vi "SaveToLVSET.vi"(6 "Save?":bool, 7 "Overwrite Existing Default Settings?":bool, 8 "Error In":errorcluster, 11 "System Paramters For Each Module":T1[](array[typedef]) {"sync_freq_div" items=["1"=1, "2"=2, "4"=4]; "cfd_zc_level" min=-96 max=96 step=0.1 format="%#_3g"; "cfd_limit_low" min=-500 max=0 step=0.1 format="%#_3g"; "sync_zc_level" min=-96 max=96 step=0.1 format="%#_3g"; "sync_threshold" min=-500 max=-20 step=0.1 format="%#_3g"; "tac_limit_low" format="%.3g"; "tac_limit_high" min=0 max=100 step=0.1 format="%.3g"; "collect_time" min=1e-07 max=100000 step=0.001; "tac_offset" min=0 max=100 step=0.1 format="%.4g"; "tac_gain" min=1 max=15 step=1; "tac_range" format="%^#_6g"}) -> (0 "Error Out":errorcluster)   [LabVIEW 2017]
doc: "This convenience VI stores the given system parameters into a LVSET file. The default file which is also used as the file to store the last used settings for each module is located in \"C:\\BHdata\\SPCM\\SPCDefaultVal.lvset\". \nThe user has the choice to overwrite this file or to use another file location to store the settings. \n\ninfo@becker-hickl.com"
uses:
  Example_Controls/UserInput.ctl
panel:
  in  "Saving Path":path=path "C:/BHdata/SPCM/SPCDefaultVal.lvset"
  # "TAC / Time Range"
  # "CFD"
  # "(start)"
  # "SYNC"
  # "(stop)"
  # "range"
  # "gain"
  # "threshold(LL)"
  # "offset"
  # "limit high"
  # "limit low"
  # "zero cross(ZC)"
  # "Collection Time"
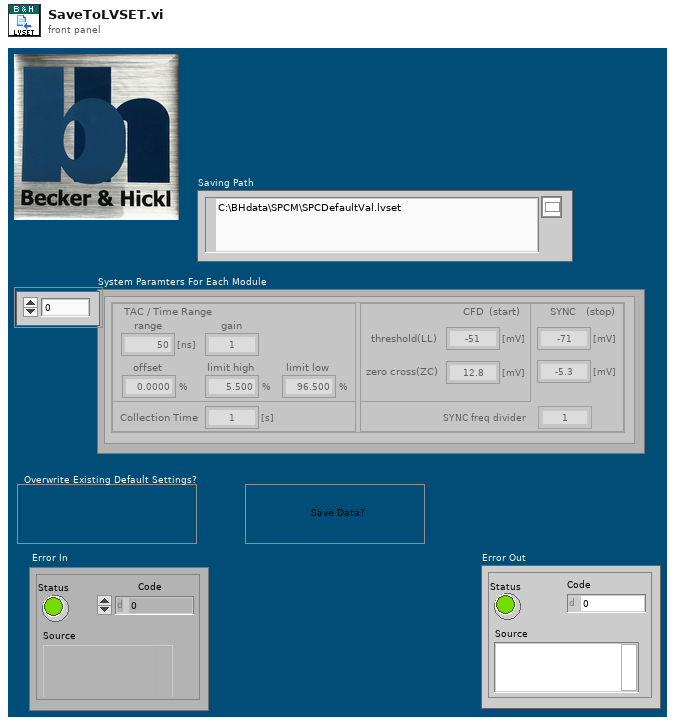
[diagram p1: front panel]
types:
  T1 = typedef "UserInput.ctl" = cluster{"tac_range":sgl, "tac_gain":i16, "tac_offset":sgl, "tac_limit_high":sgl, "tac_limit_low":sgl, "collect_time":sgl, "sync_threshold":sgl, "sync_zc_level":sgl, "sync_freq_div":i16, "cfd_limit_low":sgl, "cfd_zc_level":sgl}
  T2 = enum16{"big-endian, network order", "native, host order", "little-endian"}
  T3 = enum16{"open", "replace", "create", "open or create", "replace or create", "replace or create with confirmation"}
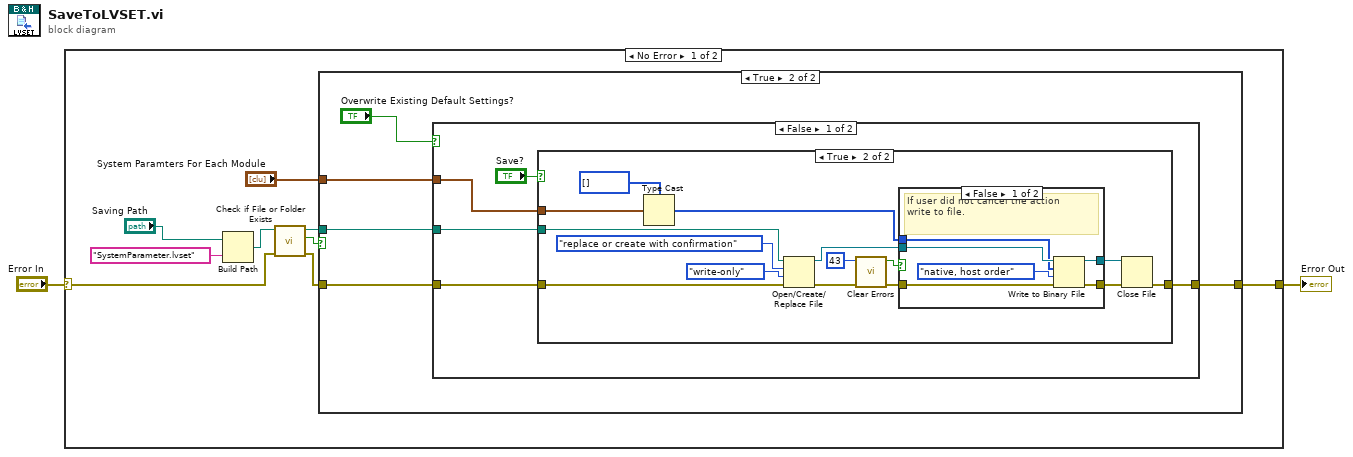
[diagram p0: block diagram]
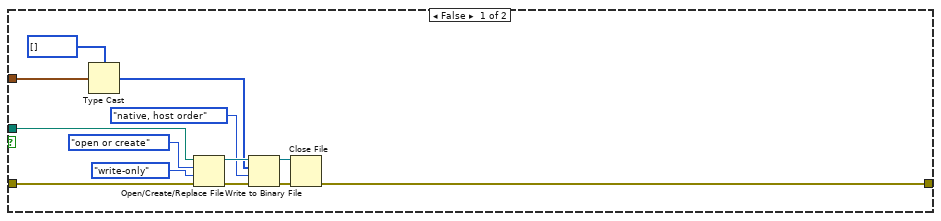
[diagram p2: hidden frame]
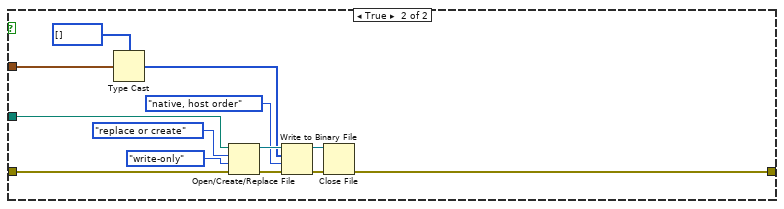
[diagram p5: hidden frame]
diagram:
  n1 = case shown="No Error" "Error In" {
    selector: "Error In" -> [w4 w72]
    tunnel: [w8 w72] -> w2
    frame No Error {
      n2 = Build Path(base path="Saving Path", name or relative path="SystemParameter.lvset") -> (appended path=w5:path)
      n3 = call <vilib>:"Check if File or Folder Exists.vi"("error in (no error)"=w4, "path"=w5) -> ("error out"=w3:errorcluster, "file or folder exists?"=w10:bool, "dup path"=w11:path)  [unwired: 7 in]
      n4 = case shown="True" w10 {
        tunnel: w11 -> [w24 w29]
        tunnel: w3 -> [w23 w28]
        tunnel: [w22 w27] -> w8
        tunnel: "System Paramters For Each Module" -> [w15 w26]
        frame False {
          n5 = Type Cast(type=u8[] [], x=w15) -> (*(type *) &x=w13:u8[])
          n6 = Open/Create/Replace File(file path (use dialog)=w24, error in=w23, operation (0:open)=T3."open or create", access (0:read/write)=enum16{"read/write", "read-only", "write-only"}."write-only") -> (refnum out=w19:refnum<file>, error out=w18:errorcluster)  [unwired: 2 in, 1 out]
          n7 = Write to Binary File(file (use dialog)=w19, data=w13, error in=w18, 9:T2."native, host order" ("byte order (0:big-endian, network order)")) -> (refnum out=w17:refnum<file>, error out=w16:errorcluster)  [unwired: 2 in, 1 out]
          n8 = Close File(refnum=w17, error in=w16) -> (error out=w22:errorcluster)  [unwired: 1 out]
        }
        frame True {
          n9 = case shown="False" "Overwrite Existing Default Settings?" {
            tunnel: w29 -> [w30 w71]
            tunnel: w28 -> [w34 w68]
            tunnel: [w32 w63] -> w27
            tunnel: w26 -> [w33 w60]
            frame False {
              n10 = case shown="True" "Save?" {
                tunnel: w34 -> [w35 w42]
                tunnel: w33 -> [_ w41]
                tunnel: [w35 w40] -> w32
                tunnel: w30 -> [_ w39]
                frame False {
                }
                frame True {
                  n11 = Type Cast(type=u8[] [], x=w41) -> (*(type *) &x=w46:u8[])
                  n12 = Open/Create/Replace File(file path (use dialog)=w39, error in=w42, operation (0:open)=T3."replace or create with confirmation", access (0:read/write)=enum16{"read/write", "read-only", "write-only"}."write-only") -> (refnum out=w50:refnum<file>, error out=w49:errorcluster)  [unwired: 2 in, 1 out]
                  n13 = call <vilib>:"Clear Errors.vi"("error in (no error)"=w49, "specific error code to clear (0: all)"=43) -> ("error out"=w38:errorcluster, "specific error cleared?"=w36:bool)  [unwired: 4 in]
                  n14 = case shown="False" w36 {
                    tunnel: w50 -> [w56 w58]
                    tunnel: w38 -> [w55 w57]
                    tunnel: [w54 w58] -> w48
                    tunnel: [w53 w57] -> w47
                    tunnel: w46 -> [w52 _]
                    frame False {
                      # "If user did not cancel the action\nwrite to file."
                      n15 = Write to Binary File(file (use dialog)=w56, data=w52, error in=w55, 9:T2."native, host order" ("byte order (0:big-endian, network order)")) -> (refnum out=w54:refnum<file>, error out=w53:errorcluster)  [unwired: 2 in, 1 out]
                    }
                    frame True {
                    }
                  }
                  n16 = Close File(refnum=w48, error in=w47) -> (error out=w40:errorcluster)  [unwired: 1 out]
                }
              }
            }
            frame True {
              n17 = Type Cast(type=u8[] [], x=w60) -> (*(type *) &x=w61:u8[])
              n18 = Open/Create/Replace File(file path (use dialog)=w71, error in=w68, operation (0:open)=T3."replace or create", access (0:read/write)=enum16{"read/write", "read-only", "write-only"}."write-only") -> (refnum out=w67:refnum<file>, error out=w66:errorcluster)  [unwired: 2 in, 1 out]
              n19 = Write to Binary File(file (use dialog)=w67, data=w61, error in=w66, 9:T2."native, host order" ("byte order (0:big-endian, network order)")) -> (refnum out=w65:refnum<file>, error out=w64:errorcluster)  [unwired: 2 in, 1 out]
              n20 = Close File(refnum=w65, error in=w64) -> (error out=w63:errorcluster)  [unwired: 1 out]
            }
          }
        }
      }
    }
    frame Error {
    }
  }
  "Error Out" <- w2
